vi "Single Panel - Insert VI - Subpanel.vi"(11 "VI Name":string) -> ()   [LabVIEW 2014]
uses:
  <vilib>/Utility/miscctls.llb/LVPositionTypeDef.ctl
  <vilib>/Utility/miscctls.llb/LVBoundsTypeDef.ctl
  VI Data.ctl
  Panel Data.ctl
  <vilib>/Utility/miscctls.llb/LVPointTypeDef.ctl
  Panel Global Methods.ctl
  Sub Function/Windows Utilities/Controls/Window Rectangle.ctl
  Sub Function/Windows Utilities/WinUtil HWND/Get Window HWnd.vi
  Sub Function/Windows Utilities/WinUtil HWND/Get Window Rectangle (hwnd).vi
  Sub Function/Windows Utilities/WinUtil HWND/Window Style/Set Window GWL_Style.vi
  <userlib>/_OpenG.lib/error/error.llb/Build Error Cluster__ogtk.vi
  Sub Function/Windows Utilities/WinUtil HWND/Window Style/Modify Window Style.vi
  <userlib>/_OpenG.lib/file/file.llb/Strip Path Extension - String__ogtk.vi
panel:
  in  "Dock Event":refnum<user-event>
  in  "Events Registered":T1
  in  "Move Event":refnum<user-event>
  in  "error in (no error)":errorcluster
  in  "Menu":bool
  in  "Pane Offset":T2={"Left"=0, "Top"=22}
  in  "User Events VR":variant
  out "error out":errorcluster
  in  "Title":string
  in  "Undock":bool
  in  "Expand":bool
  in  "Containing Pane":refnum<vi>
  out "2D Picture":picture
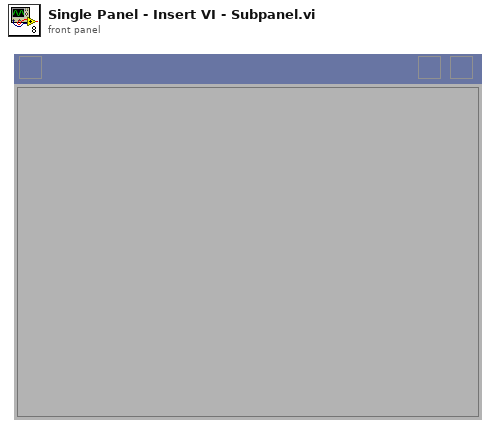
[diagram p1: front panel]
types:
  T1 = typedef "Semaphore RefNum" = refnum<k1>
  T2 = typedef "LVPositionTypeDef.ctl" = cluster{"Left":i32, "Top":i32}
  T3 = typedef "Panel Data.ctl" = cluster{"Panel VI Name":string, "Hwnd":u32, "Collapsed?":bool, "Panel Ref":refnum<vi>, "Events Variant":variant, "Resizeable?":bool, "Un-Dockedable?":bool, "Docked?":bool}
  T4 = typedef "VI Data.ctl" = cluster{"VI Name":string, "VI Ref":refnum<vi>, "Events Variant":variant, "Panel Settings":variant}
  T5 = typedef "LVBoundsTypeDef.ctl" = cluster{"Width":u32, "Height":u32}
  T6 = cluster{"Event Ref":refnum<event-registration>, "Reposition Offset":cluster{"Left":i16, "Top":i32}, "Saved Panel Size":T5, "Sub Panel":refnum<vi>, "VI Data":T4, "Panel Data":T3, "Reply User Event":refnum<user-event>, "Parent Hwnd":u32, "Parent Pane":refnum<vi>, "Pane Offset":T2, "Currently Resizeable?":bool, "Move Event":refnum<user-event>, "Dock Event":refnum<user-event>}
  T7 = typedef "LVPointTypeDef.ctl" = cluster{"Horizontal":i16, "Vertical":i16}
  T8 = enum8{"Enabled", "Disabled", "Disabled and Grayed Out"}
  T9 = typedef "Panel Global Methods.ctl" = enum16{"Read All Panels", "Read Panel Data", "Write Panel Data"}
  T10 = typedef "Window Rectangle.ctl" = cluster{"left":i16, "top":i16, "right":i16, "bottom":i16}
  T11 = enum16{"Clear Error And Continue", "Notify User Clear Error", "Clear Error Cleanup"}
  T12 = typedef "LVRectTypeDef.ctl" = cluster{"Left":i16, "Top":i16, "Right":i16, "Bottom":i16}
  T13 = typedef "Window Rectangle (hwnd).ctl" = cluster{"left":i16, "top":i16, "right":i16, "bottom":i16}
  T14 = typedef "imagedata.ctl" = cluster{"image type":i32, "image depth":i32, "image":u8[], "mask":u8[], "colors":u32[], "Rectangle":cluster{"left":i16, "top":i16, "right":i16, "bottom":i16}}
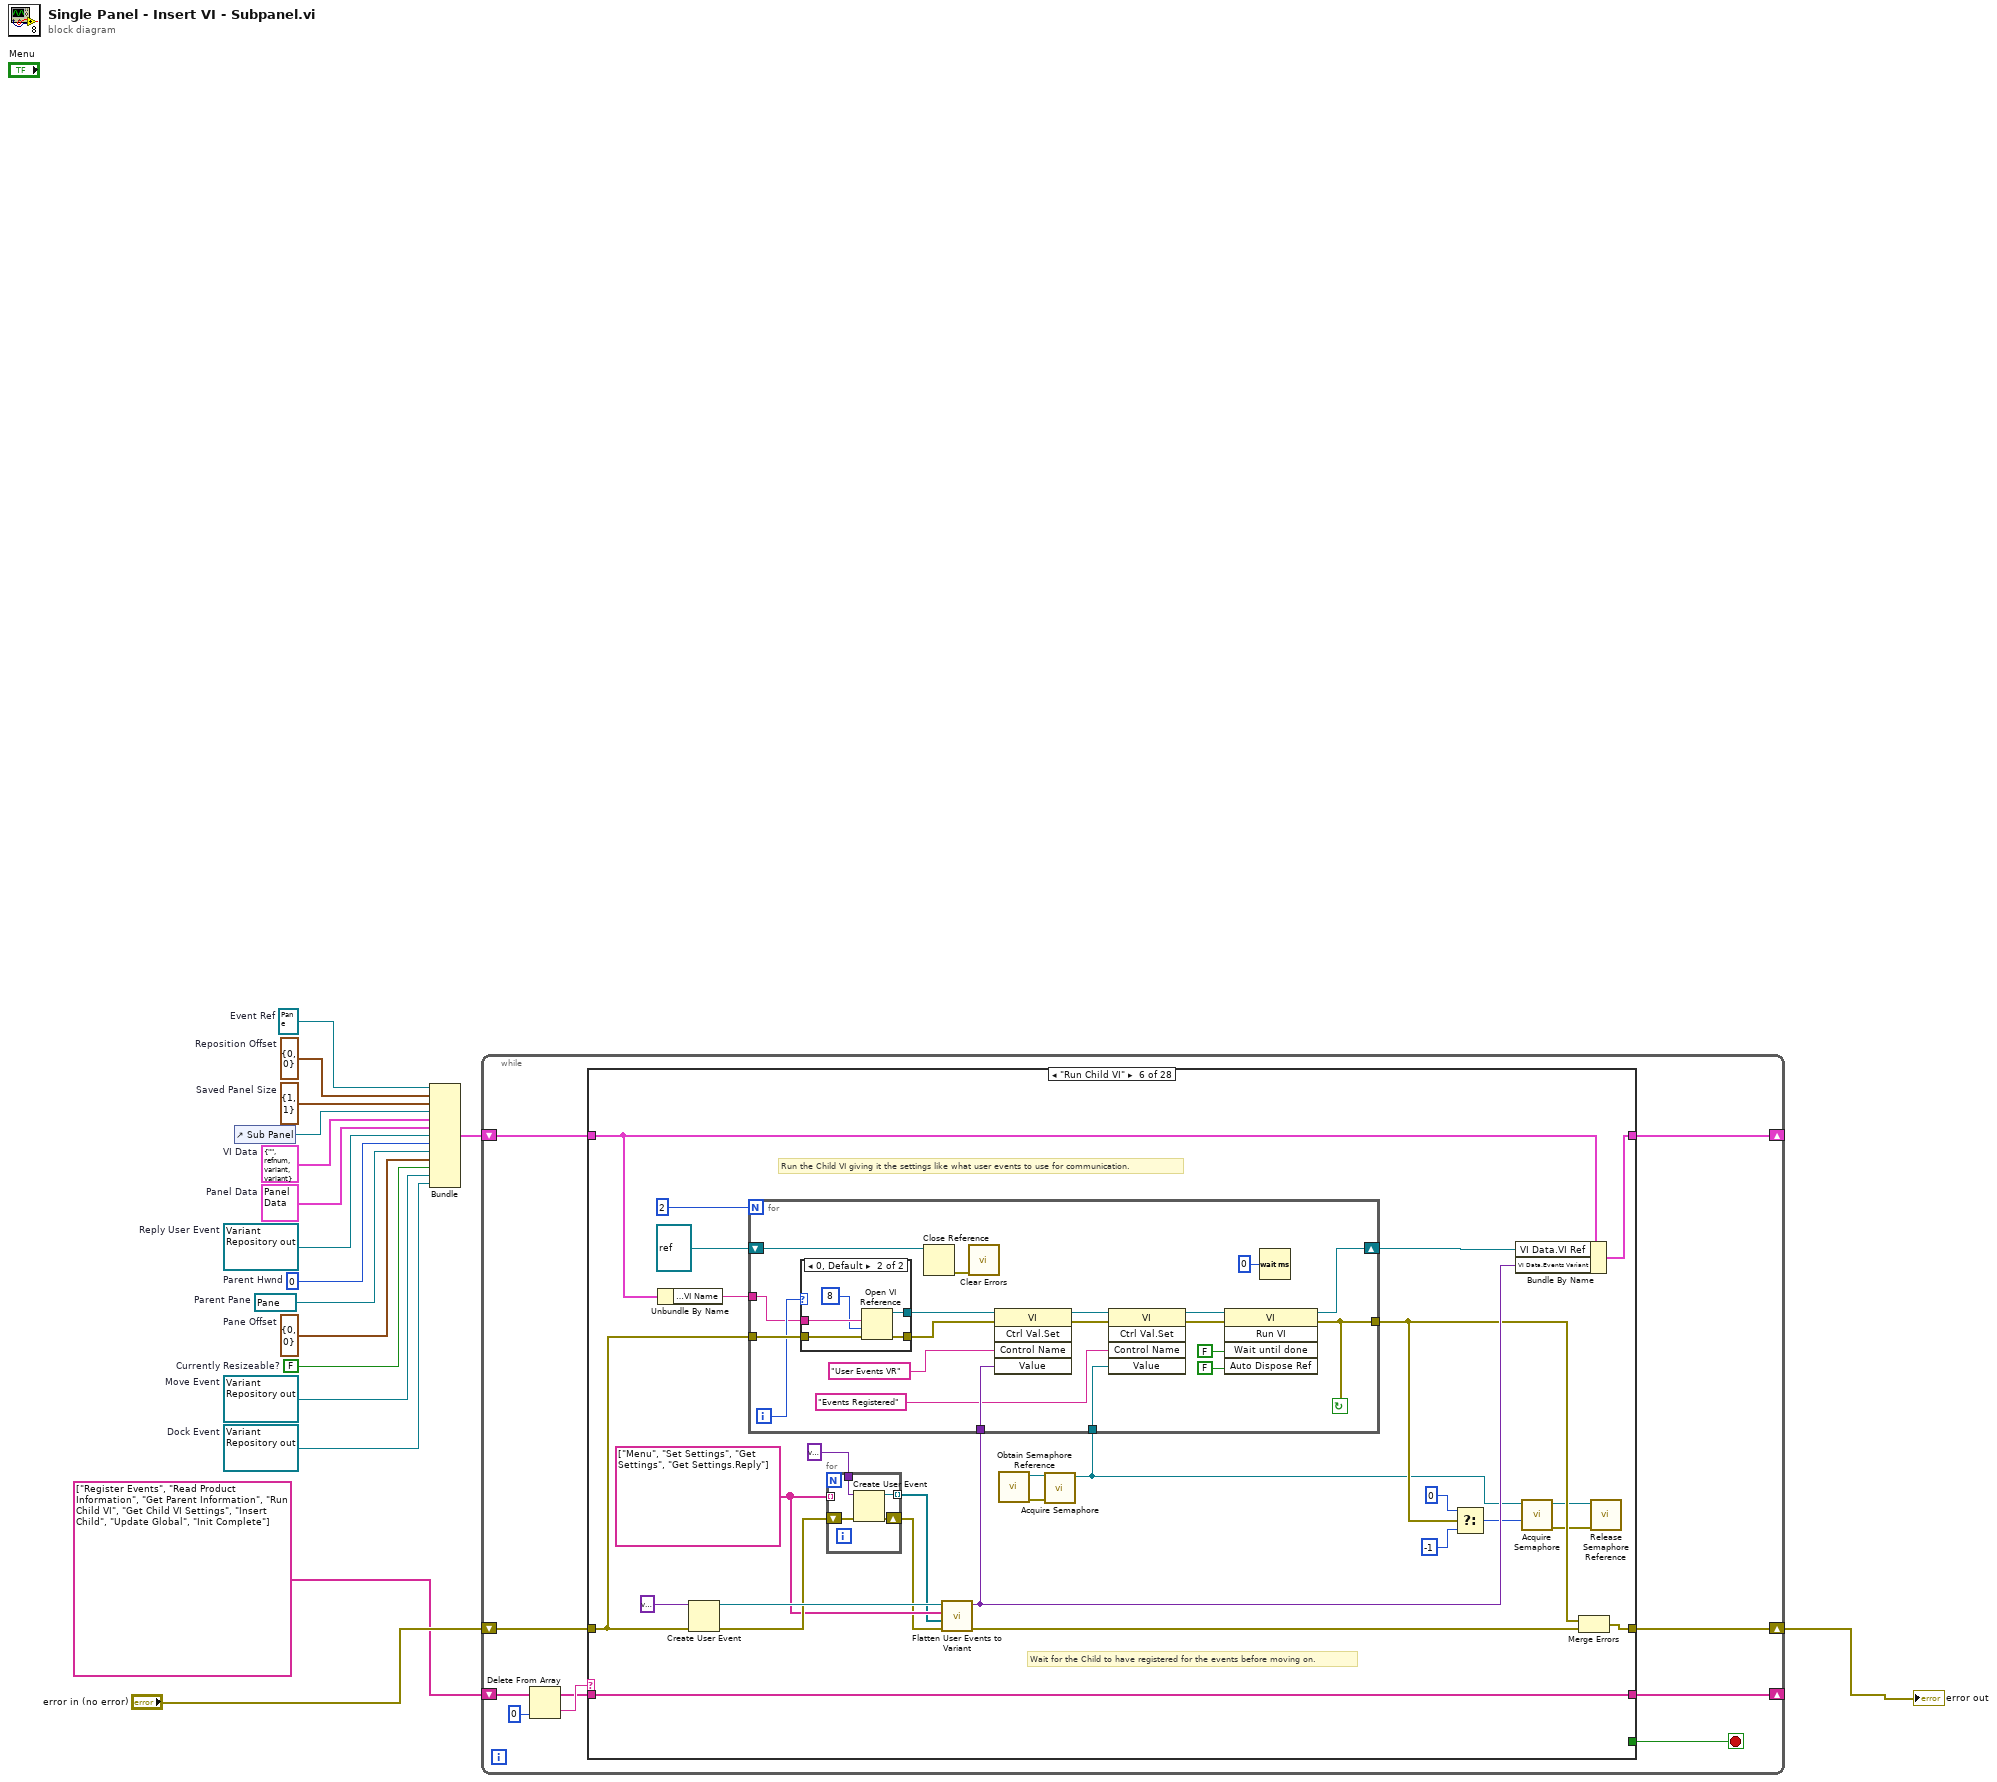
[diagram p0: block diagram]
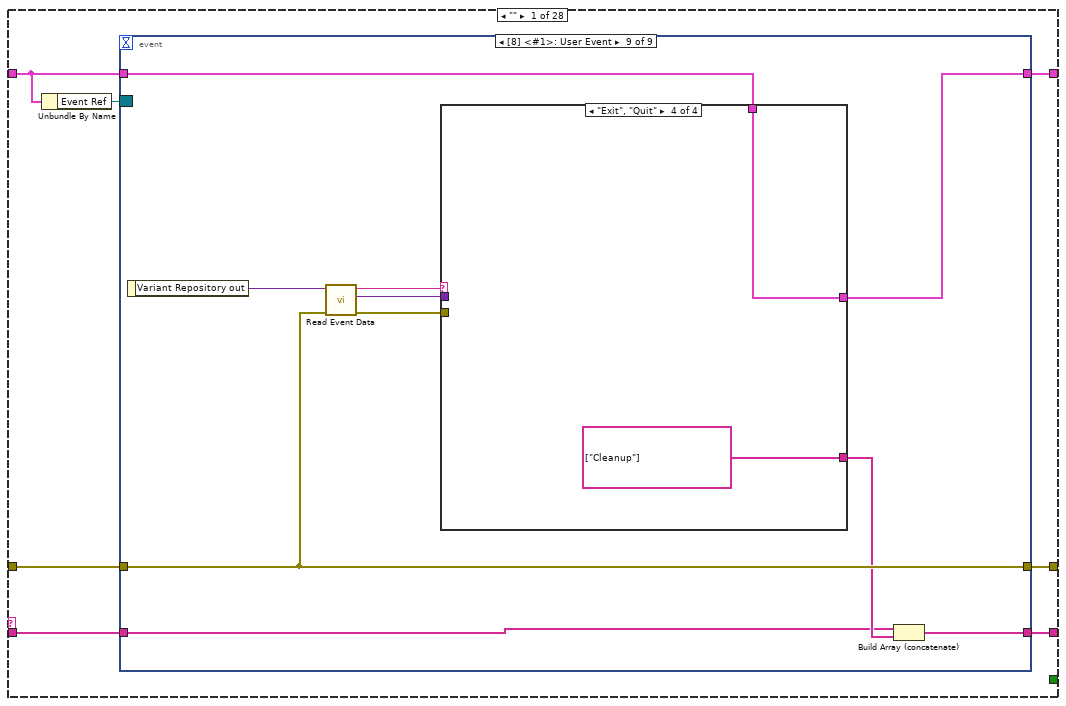
[diagram p2: hidden frame]
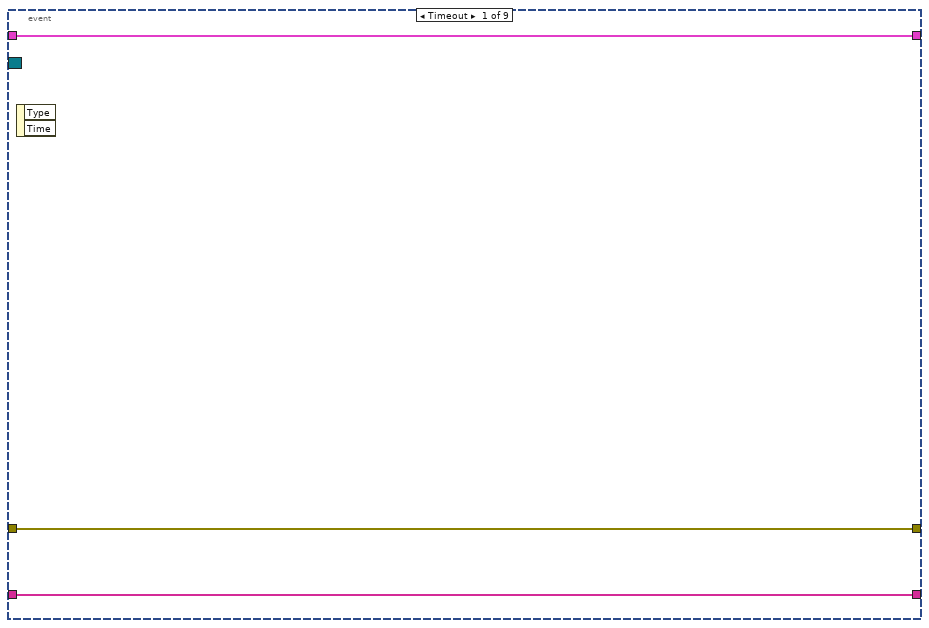
[diagram p3: hidden frame]
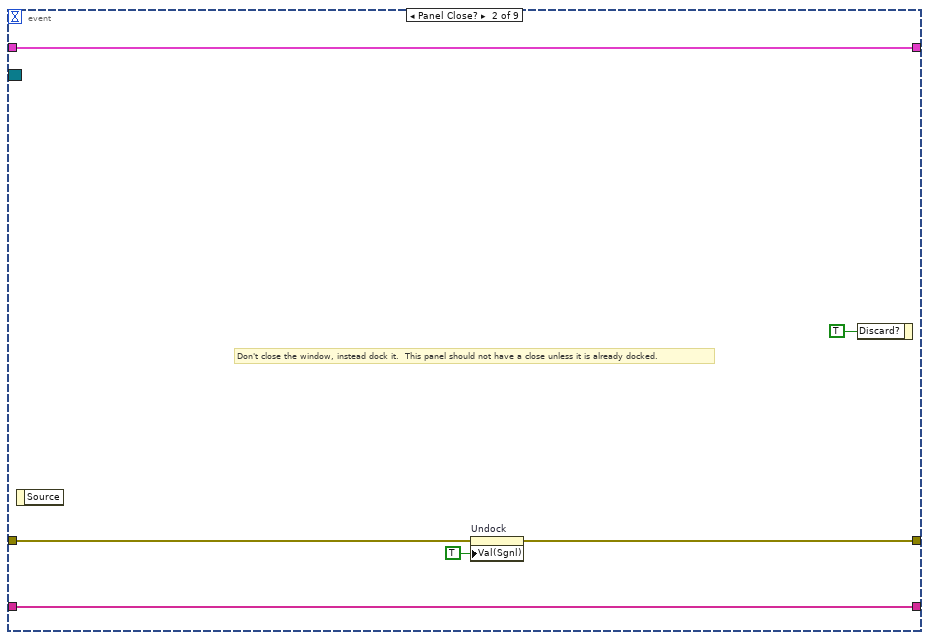
[diagram p4: hidden frame]
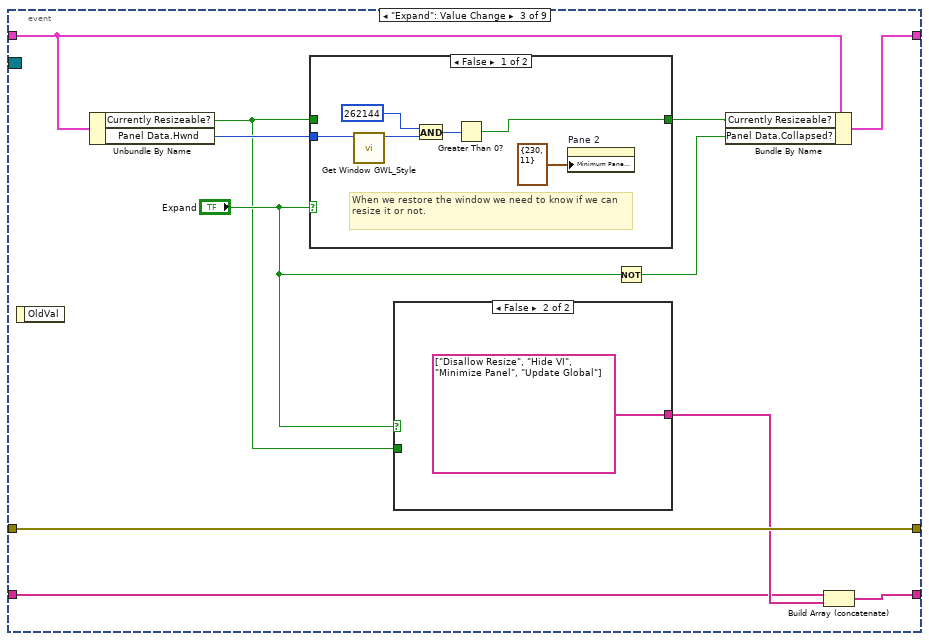
[diagram p5: hidden frame]
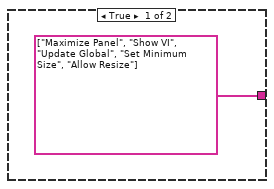
[diagram p6: hidden frame]
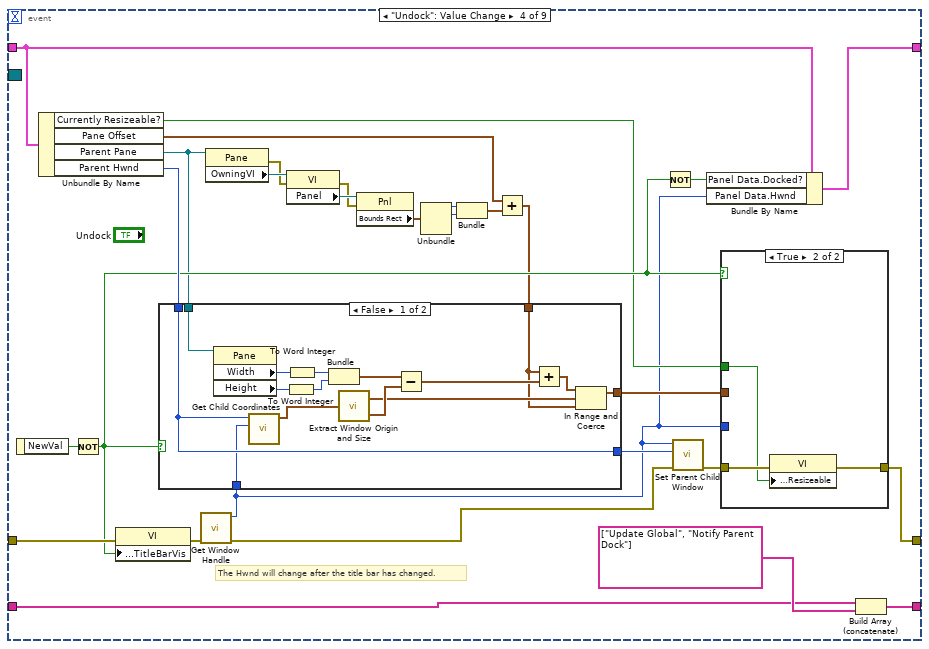
[diagram p8: hidden frame]
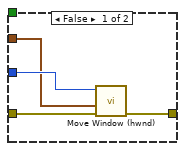
[diagram p9: hidden frame]
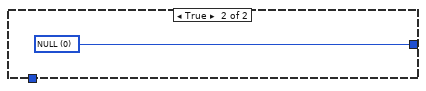
[diagram p10: hidden frame]
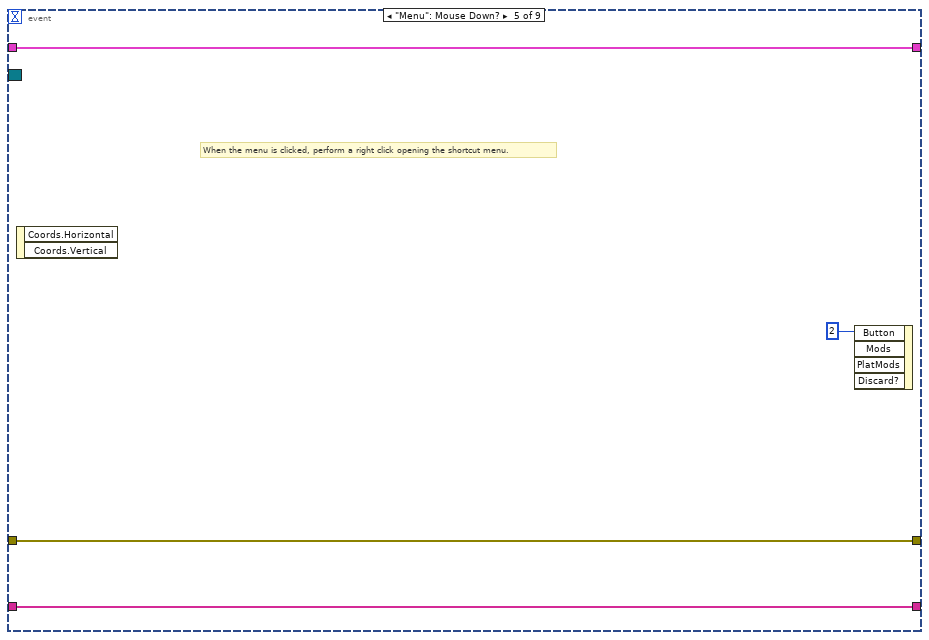
[diagram p11: hidden frame]
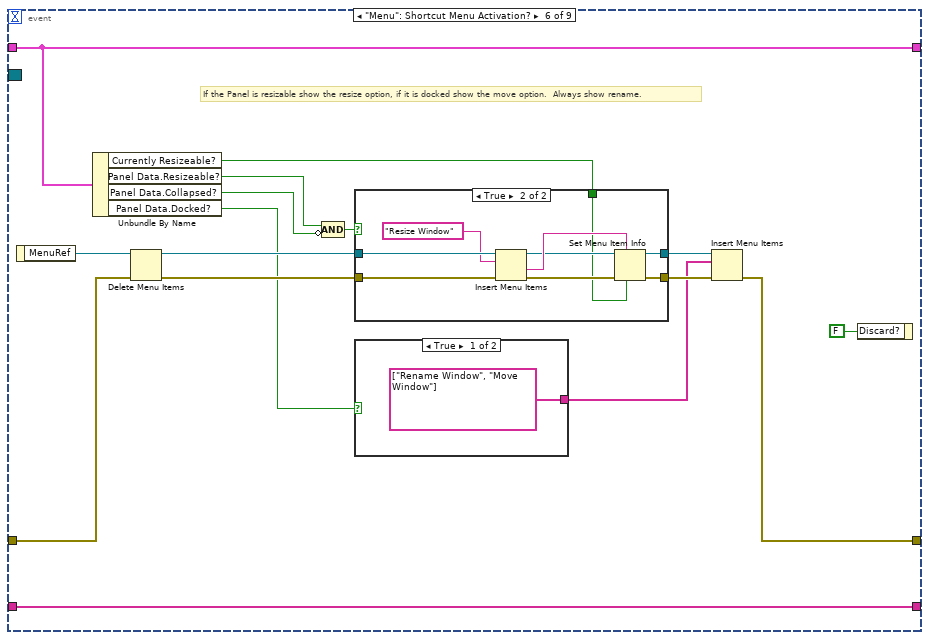
[diagram p12: hidden frame]
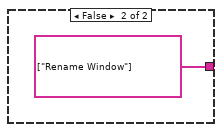
[diagram p13: hidden frame]
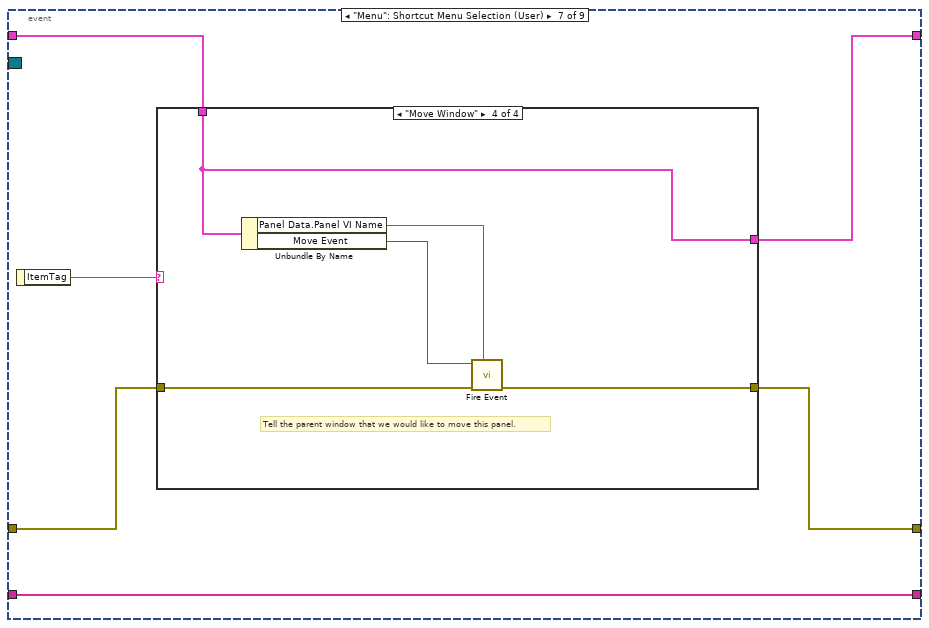
[diagram p15: hidden frame]
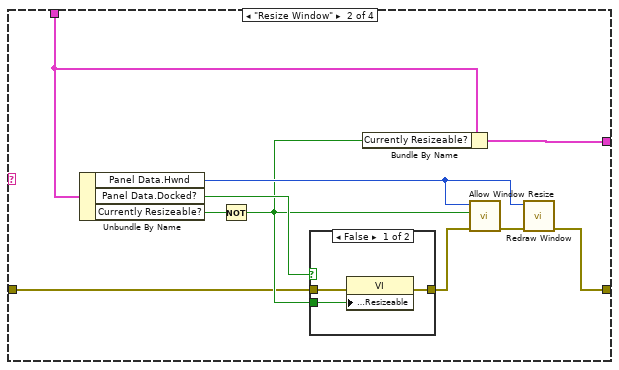
[diagram p17: hidden frame]
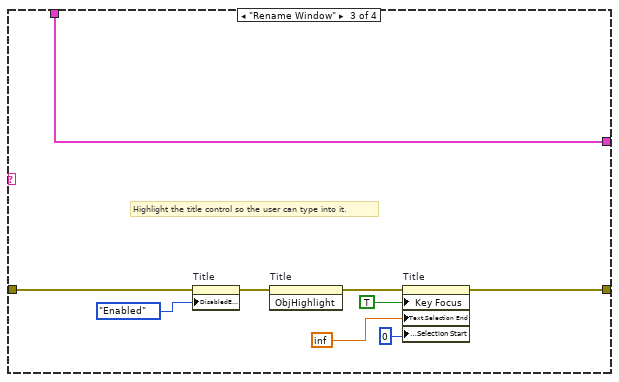
[diagram p19: hidden frame]
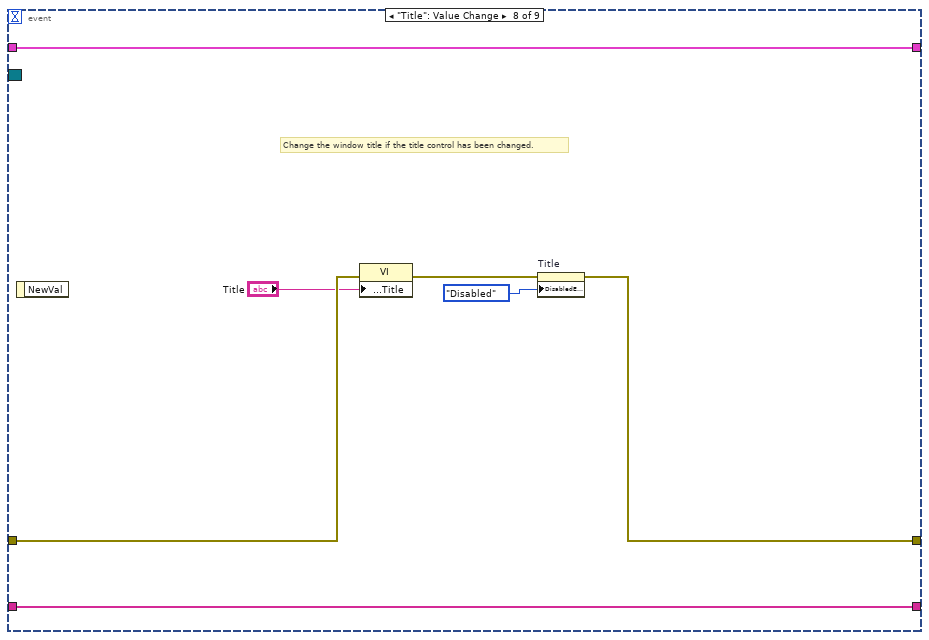
[diagram p20: hidden frame]
diagram:
  w3 = refnum<user-event> refnum  # Dock Event
  w4 = refnum<user-event> refnum  # Move Event
  w5 = FALSE  # Currently Resizeable?
  w6 = T2 {"Left"=0, "Top"=0}  # Pane Offset
  w7 = refnum<vi> refnum  # Parent Pane
  w8 = u32 0  # Parent Hwnd
  w9 = refnum<user-event> refnum  # Reply User Event
  w10 = refnum<event-registration> refnum  # Event Ref
  w11 = T3 {"Panel VI Name"="", "Hwnd"=0, "Collapsed?"=FALSE, "Panel Ref"=refnum, "Events Variant"=variant, "Resizeable?"=FALSE, "Un-Dockedable?"=FALSE, "Docked?"=FALSE}  # Panel Data
  w12 = T4 {"VI Name"="", "VI Ref"=refnum, "Events Variant"=variant, "Panel Settings"=variant}  # VI Data
  w14 = T5 {"Width"=1, "Height"=1}  # Saved Panel Size
  w15 = cluster{"Left":i16, "Top":i32} {"Left"=0, "Top"=0}  # Reposition Offset
  n1 = control-ref of="Sub Panel"() -> (w13:refnum<vi>)
  n2 = Bundle("Event Ref"=w10, "Reposition Offset"=w15, "Saved Panel Size"=w14, "Sub Panel"=w13, "VI Data"=w12, "Panel Data"=w11, "Reply User Event"=w9, "Parent Hwnd"=w8, "Parent Pane"=w7, "Pane Offset"=w6, "Currently Resizeable?"=w5, "Move Event"=w4, "Dock Event"=w3) -> (w17:T6)  [unwired: 1 in]
  n3 = while {
    shift-right: [w23] -> w2
    shift-left: "error in (no error)" -> [w27]
    shift-right: [w25] -> _
    shift-left: w17 -> [w26]
    shift-right: [w18] -> _
    shift-left: string[] ["Register Events", "Read Product Information", "Get Parent Information", "Run Child VI", "Get Child VI Settings", "Insert Child", "Update Global", "Init Complete"] ("Initialized States") -> [w19]
    stop <- w24 stop-if-true
    n4 = Delete From Array(array=w19, index=0) -> (deleted portion=w21:string, array with subset deleted=w20:string[])  [unwired: 1 in]
    n5 = case "State Machine" shown="\"Run Child VI\"" w21 {
      selector: w21 -> [_ _ _ _ _ _ _ _ _ _ _ _ _ _ _ _ w466 w477 _ _ _ _ w589 _ _ _ _ _]
      tunnel: w20 -> [w34 w212 w244 w263 w282 w309 w344 w367 w376 w394 w402 w404 w419 w426 w447 w457 w470 w481 w548 w555 w567 w569 w593 w596 w598 w611 w616 w620]
      tunnel: [w30 w212 w244 w263 w282 w309 w343 w367 w376 w394 w402 w403 w419 w426 w447 w457 w470 w481 w548 w555 w567 w570 w593 w596 w597 w611 w616 w620] -> w18
      tunnel: [w31 w210 w232 w247 w266 w303 w350 w356 w372 w377 w396 w408 w418 w425 w431 w448 w462 w506 w544 w550 w566 w571 w586 w595 w601 w603 w612 w617] -> w23
      tunnel: w27 -> [w32 w210 w226 w248 w264 w290 w351 w357 w375 w387 w397 w409 w418 w422 w435 w450 w460 w506 w545 w551 w566 w572 w587 w595 w601 w605 w613 w617]
      tunnel: w26 -> [w29 w211 w243 w262 w281 w305 w355 w366 w374 w393 w401 w411 w417 w423 w446 w454 w468 w476 w547 w552 w565 w573 w592 w594 w600 w608 w615 w619]
      tunnel: [w33 w211 w234 w257 w277 w306 w354 w366 w374 w383 w401 w407 w417 w423 w446 w452 w468 w475 w547 w552 w565 w573 w592 w594 w600 w608 w615 w619] -> w25
      tunnel: [_ _ _ _ _ _ _ _ _ _ _ _ _ _ _ _ _ _ _ _ _ _ _ _ _ _ _ TRUE] -> w24
      frame "" {
        n6 = Unbundle By Name(w29) -> ("Event Ref"=w28:refnum<event-registration>)
        n7 = event shown="[8] <#1>: User Event" {
          selector: w28 -> [_ _ _ _ _ _ _ _ _]
          dyn-events: _ -> [_ _ _ _ _ _ _ _ _]
          timeout: _ -> [_ _ _ _ _ _ _ _ _]
          tunnel: w29 -> [w37 w41 w52 w92 w119 w130 w151 w188 w195]
          tunnel: w34 -> [w35 w42 w45 w65 w117 w135 w154 w190 w192]
          tunnel: [w37 w41 w53 w85 w119 w130 w153 w188 w194] -> w33
          tunnel: w32 -> [w36 w39 w54 w91 w118 w122 w150 w186 w199]
          tunnel: [w36 w38 w54 w84 w118 w121 w149 w185 w199] -> w31
          tunnel: [w35 w42 w44 w64 w117 w135 w154 w190 w191] -> w30
          event Timeout {
            n8 = event-data() -> ()  [unwired: 1 in, 2 out]
          }
          event Panel Close? {
            # "Don't close the window, instead dock it.  This panel should not have a close unless it is already docked."
            n9 = event-data() -> ()  [unwired: 1 in, 1 out]
            n10 = property on="Undock" class="Bool (strict)"(error in=w39, "Val(Sgnl)"=TRUE ("Value (Signaling)")) -> (error out=w38:errorcluster)  [unwired: 1 in, 1 out]
            n11 = event-data("Discard?"=TRUE) -> ()  [unwired: 1 in, 1 out]
          }
          event "Expand": Value Change {
            n12 = event-data() -> ()  [unwired: 1 in, 1 out]
            n13 = Unbundle By Name(w52) -> ("Currently Resizeable?"=w47:bool, "Panel Data.Hwnd"=w50:u32)
            n14 = case shown="False" "Expand" {
              tunnel: w50 -> [w61 _]
              tunnel: [w57 w63] -> w49
              tunnel: w47 -> [_ w63]
              frame False {
                # "When we restore the window we need to know if we can resize it or not."
                n15 = call "Get Window GWL_Style.vi"("Hwnd"=w61) -> ("Style"=w60:u32)  [unwired: 9 in, 1 out]
                n16 = And(x=u32 262144 ("Value"), y=w60) -> (x .and. y?=w58:u32)
                n17 = Greater Than 0?(x=w58) -> (x > 0?=w57:bool)
                n18 = property on="Pane 2" class="Pane"("Minimum Pane Size"=T7 {"Horizontal"=230, "Vertical"=11}) -> ()  [unwired: 2 in, 2 out]
              }
              frame True {
              }
            }
            n19 = case shown="False" "Expand" {
              tunnel: [string[] ["Maximize Panel", "Show VI", "Update Global", "Set Minimum Size", "Allow Resize"] ("Elements to Add") string[] ["Disallow Resize", "Hide VI", "Minimize Panel", "Update Global"] ("Elements to Add")] -> w46
              tunnel: w47 -> [_ _]
              frame True {
              }
              frame False {
              }
            }
            n20 = Not(x="Expand") -> (.not. x?=w48:bool)
            n21 = Bundle By Name(cluster=w52, "Currently Resizeable?"=w49, "Panel Data.Collapsed?"=w48) -> (w53:T6)
            n22 = Build Array (concatenate)(w45, w46) -> (w44:string[])
          }
          event "Undock": Value Change {
            # "The Hwnd will change after the title bar has changed."
            n23 = event-data() -> ("NewVal"=w88:bool)  [unwired: 1 in]
            n24 = Unbundle By Name(w92) -> ("Currently Resizeable?"=w79:bool, "Pane Offset"=w71:T2, "Parent Pane"=w78:refnum<vi>, "Parent Hwnd"=w89:u32)
            n25 = Not(x=w88) -> (.not. x?=w82:bool)
            n26 = property class="VI"(error in=w91, "Front Panel.TitleBarVis"=w82) -> (error out=w87:errorcluster)  [unwired: 1 in, 1 out]
            n27 = call "Get Window Handle.vi"("error in (no error)"=w87) -> ("error out"=w86:errorcluster, "HWnd Out"=w67:u32)  [unwired: 9 in]
            n28 = property class="Pane"(reference=w78) -> (error out=w69:errorcluster, "OwningVI"=w77:refnum<vi>)  [unwired: 1 in, 1 out]
            n29 = property class="VI"(reference=w77, error in=w69) -> (error out=w68:errorcluster, "Panel"=w76:refnum<vi>)  [unwired: 1 out]
            n30 = property class="Pnl"(reference=w76, error in=w68) -> ("Bounds Rect"=w75:T12)  [unwired: 2 out]
            n31 = Unbundle(w75) -> ("Left"=w74:i16, "Top"=w73:i16)  [unwired: 2 out]
            n32 = Bundle("Left"=w74, "Top"=w73) -> (w72:cluster{"Left":i16, "Top":i16})  [unwired: 1 in]
            n33 = Add(x=w71, y=w72) -> (x+y=w70:T2)
            n34 = case shown="False" w82 {
              tunnel: [w111 w115] -> w80
              tunnel: w89 -> [w111 _]
              tunnel: [w104 _] -> w83
              tunnel: w67 -> [w110 _]
              tunnel: w78 -> [w109 _]
              tunnel: w70 -> [w100 _]
              frame False {
                n35 = property class="Pane"(reference=w109) -> ("Width"=w108:u32, "Height"=w107:u32)  [unwired: 1 in, 2 out]
                n36 = call "Get Child Coordinates.vi"("Child hWnd"=w110, "Parent hWnd"=w111) -> ("Relative"=w114:T13)  [unwired: 7 in, 2 out]
                n37 = To Word Integer(number=w107) -> (16bit integer=w102:i16)
                n38 = To Word Integer(number=w108) -> (16bit integer=w103:i16)
                n39 = Bundle(w103, w102) -> (w112:cluster{i16, i16})  [unwired: 1 in]
                n40 = call "Extract Window Origin and Size.vi"("window rect"=w114) -> ("window origin"=w106:cluster{"left":i16, "top":i16}, "window size"=w113:cluster{"width":i16, "height":i16})
                n41 = Subtract(x=w112, y=w113) -> (x-y=w105:cluster{i16, i16})
                n42 = Add(x=w100, y=w105) -> (x+y=w101:T2)
                n43 = In Range and Coerce(upper limit=w101, x=w106, lower limit=w100) -> (coerced(x)=w104:T2)  [unwired: 1 out]
              }
              frame True {
                w115 = u32 0 items=["NULL"]
              }
            }
            n44 = Not(x=w82) -> (.not. x?=w81:bool)
            n45 = call "Set Parent Child Window.vi"("error in (no error)"=w86, "new parent"=w80, "child"=w67) -> ("error out"=w90:errorcluster)  [unwired: 8 in]
            n46 = Bundle By Name(cluster=w92, "Panel Data.Docked?"=w81, "Panel Data.Hwnd"=w67) -> (w85:T6)
            n47 = case shown="True" w82 {
              tunnel: w90 -> [w96 w99]
              tunnel: [w95 w98] -> w84
              tunnel: w67 -> [w94 _]
              tunnel: w83 -> [w93 _]
              tunnel: w79 -> [_ w97]
              frame False {
                n48 = call "Move Window (hwnd).vi"("error in (no error)"=w96, "New Position (0,0)"=w93, "HWnd"=w94) -> ("error out"=w95:errorcluster)  [unwired: 6 in, 2 out]
              }
              frame True {
                n49 = property class="VI"(error in=w99, "Front Panel.Resizeable"=w97) -> (error out=w98:errorcluster)  [unwired: 1 in, 1 out]
              }
            }
            n50 = Build Array (concatenate)(w65, string[] ["Update Global", "Notify Parent Dock"]) -> (w64:string[])
          }
          event "Menu": Mouse Down? {
            # "When the menu is clicked, perform a right click opening the shortcut menu."
            n51 = event-data() -> ()  [unwired: 1 in, 2 out]
            n52 = event-data("Button"=u16 2) -> ()  [unwired: 4 in, 1 out]
          }
          event "Menu": Shortcut Menu Activation? {
            # "If the Panel is resizable show the resize option, if it is docked show the move option.  Always show rename."
            n53 = event-data() -> ("MenuRef"=w134:refnum<k9>)  [unwired: 1 in]
            n54 = Unbundle By Name(w130) -> ("Currently Resizeable?"=w129:bool, "Panel Data.Resizeable?"=w128:bool, "Panel Data.Collapsed?"=w126:bool, "Panel Data.Docked?"=w120:bool)
            n55 = Delete Menu Items(6:w122, 9:w134) -> (0:w132:errorcluster, 3:w133:refnum<k9>)  [unwired: 2 in]
            n56 = Compound Arithmetic op=AND(w128, invert w126) -> (w127:bool)
            n57 = case shown="True" w127 {
              tunnel: w133 -> [w139 w148]
              tunnel: w132 -> [w138 w147]
              tunnel: w129 -> [_ w142]
              tunnel: [w138 w141] -> w125
              tunnel: [w139 w140] -> w124
              frame False {
              }
              frame True {
                n58 = Insert Menu Items(6:w147, 8:"Resize Window", 9:w148) -> (0:w144:errorcluster, 1:w145:string, 3:w143:refnum<k9>)  [unwired: 3 in]
                n59 = Set Menu Item Info(6:w142, 7:w145, 8:w144, 11:w143) -> (0:w141:errorcluster, 3:w140:refnum<k9>)  [unwired: 3 in]
              }
            }
            n60 = case shown="True" w120 {
              tunnel: [string[] ["Rename Window", "Move Window"] string[] ["Rename Window"]] -> w123
              frame True {
              }
              frame False {
              }
            }
            n61 = Insert Menu Items(6:w125, 8:w123, 9:w124) -> (0:w121:errorcluster)  [unwired: 3 in, 2 out]
            n62 = event-data("Discard?"=FALSE) -> ()  [unwired: 1 in, 1 out]
          }
          event "Menu": Shortcut Menu Selection (User) {
            n63 = event-data() -> ("ItemTag"=w152:string)  [unwired: 1 in]
            n64 = case shown="\"Move Window\"" w152 {
              tunnel: [w156 w162 w172 w179] -> w153
              tunnel: w151 -> [w156 w159 w172 w179]
              tunnel: w150 -> [w155 w158 w171 w181]
              tunnel: [w155 w157 w170 w180] -> w149
              frame Default {
              }
              frame "Resize Window" {
                n65 = Unbundle By Name(w159) -> ("Panel Data.Hwnd"=w165:u32, "Panel Data.Docked?"=w163:bool, "Currently Resizeable?"=w161:bool)
                n66 = Not(x=w161) -> (.not. x?=w160:bool)
                n67 = case shown="False" w163 {
                  tunnel: [w169 _] -> w164
                  tunnel: w160 -> [w168 _]
                  tunnel: w158 -> [w167 _]
                  frame False {
                    n68 = property class="VI"(error in=w167, "Front Panel.Resizeable"=w168) -> (error out=w169:errorcluster)  [unwired: 1 in, 1 out]
                  }
                  frame True {
                  }
                }
                n69 = Bundle By Name(cluster=w159, "Currently Resizeable?"=w160) -> (w162:T6)
                n70 = call "Allow Window Resize.vi"("error in (no error)"=w164, "Allow Resize?"=w160, "Hwnd"=w165) -> ("error out"=w166:errorcluster)  [unwired: 8 in]
                n71 = call "Redraw Window.vi"("error in (no error)"=w166, "Hwnd"=w165) -> ("error out"=w157:errorcluster)  [unwired: 9 in]
              }
              frame "Rename Window" {
                # "Highlight the title control so the user can type into it."
                n72 = property on="Title" class="Str"(error in=w171, "DisabledEnum"=T8."Enabled" ("Disabled")) -> (error out=w176:errorcluster)  [unwired: 1 in, 1 out]
                n73 = invoke on="Title" class="Str" method="ObjHighlight"(error in=w176) -> (error out=w175:errorcluster)  [unwired: 2 in, 2 out]
                n74 = property on="Title" class="Str"(error in=w175, "Key Focus"=TRUE, "Text.Selection End"=inf, "Text.Selection Start"=u32 0 ("Text.Selection:Start")) -> (error out=w170:errorcluster)  [unwired: 1 in, 1 out]
              }
              frame "Move Window" {
                # "Tell the parent window that we would like to move this panel."
                n75 = Unbundle By Name(w179) -> ("Panel Data.Panel VI Name"=w182:string, "Move Event"=w183:refnum<user-event>)
                n76 = call "Fire Event.vi"("Event Name"=w182, "error in (no error)"=w181, "User Event In"=w183) -> ("error out"=w180:errorcluster)  [unwired: 7 in, 1 out]
              }
            }
          }
          event "Title": Value Change {
            # "Change the window title if the title control has been changed."
            n77 = event-data() -> ()  [unwired: 1 in, 1 out]
            n78 = property class="VI"(error in=w186, "Front Panel.Title"="Title") -> (error out=w187:errorcluster)  [unwired: 1 in, 1 out]
            n79 = property on="Title" class="Str"(error in=w187, "DisabledEnum"=T8."Disabled" ("Disabled")) -> (error out=w185:errorcluster)  [unwired: 1 in, 1 out]
          }
          event User Event {
            n80 = event-data() -> ("Variant Repository out"=w200:variant)  [unwired: 1 in]
            n81 = call "Read Event Data.vi"("error in (no error)"=w199, "Variant Data"=w200) -> ("error out"=w198:errorcluster, "Event Data"=w196:variant, "Event Name"=w197:string)  [unwired: 7 in]
            n82 = case shown="\"Exit\", \"Quit\"" w197 {
              tunnel: w198 -> [_ _ _ _]
              tunnel: [_ string[] ["Get Settings", "Send Settings to Parent"] string[] ["Set Settings"] string[] ["Cleanup"]] -> w193
              tunnel: w196 -> [_ _ w204 _]
              tunnel: w195 -> [w201 w202 w206 w208]
              tunnel: [w201 w202 w205 w208] -> w194
              frame Default {
              }
              frame "Get Settings" {
              }
              frame "Set Settings" {
                n83 = Bundle By Name(cluster=w206, "VI Data.Panel Settings"=w204) -> (w205:T6)
              }
              frame "Exit", "Quit" {
              }
            }
            n84 = Build Array (concatenate)(w192, w193) -> (w191:string[])
          }
        }
      }
      frame "----Initialize----" {
      }
      frame "Register Events" {
        n85 = Get Variant Attribute(Variant="User Events VR", name="Event Names" ("Tag"), default value (empty Variant)=string[] [], error in=w226) -> (duplicate Variant=w221:variant, value=w222:string[], error out=w220:errorcluster)  [unwired: 1 out]
        n86 = Get Variant Attribute(Variant=w221, name="User Events" ("Tag"), error in=w220) -> (duplicate Variant=w217:variant, value=w218:variant, error out=w216:errorcluster)  [unwired: 1 in, 1 out]
        n87 = Search 1D Array(1D array=w222, element="Get Settings.Reply") -> (index of element=w239:i32)  [unwired: 1 in]
        n88 = Get Variant Attribute(Variant=w217, name="Quit Event" ("Tag"), error in=w216) -> (value=w214:variant, error out=w213:errorcluster)  [unwired: 1 in, 2 out]
        n89 = Variant To Data(error in=w213, type=refnum<user-event>[] [] ("All User Events"), Variant=w218) -> (data=w238:refnum<user-event>[], error out=w229:errorcluster)
        n90 = Delete From Array(array=w238, index=w239) -> (deleted portion=w231:refnum<user-event>, array with subset deleted=w237:refnum<user-event>[])  [unwired: 1 in]
        n91 = Variant To Data(error in=w229, type=refnum<user-event> refnum ("Quit Event"), Variant=w214) -> (data=w236:refnum<user-event>, error out=w228:errorcluster)
        n92 = Build Array (concatenate)(w237, w236) -> (w235:refnum<user-event>[])
        n93 = register-events(error in=w228, w235) -> (reference out=w233:refnum<event-registration>, error out=w232:errorcluster)  [unwired: 1 in]
        n94 = Bundle By Name(cluster=w243, "Dock Event"="Dock Event", "Move Event"="Move Event", "Reply User Event"=w231, "Event Ref"=w233, "Panel Data.Events Variant"="User Events VR") -> (w234:T6)
      }
      frame "Read Product Information" {
        # "Get the name of the VI to be inserted in the subpanel.  If blank just use the Graph Panel which at the moment is the only one we have."
        n95 = property on="2D Picture" class="Pict"("Visible"=FALSE) -> ()  [unwired: 2 in, 2 out]
        n96 = local write "Undock"(TRUE ("Undock")) -> ()
        n97 = property on="Pane 2" class="Pane"("PaneColor"=u32 11776947) -> ()  [unwired: 2 in, 2 out]
        n98 = local write "Expand"(TRUE ("Expand")) -> ()
        n99 = vi-ref "Graph Child.vi"() -> (w261:refnum<vi>)
        n100 = property on="Title" class="Str"("DisabledEnum"=T8."Disabled" ("Disabled")) -> ()  [unwired: 2 in, 2 out]
        n101 = property class="VI"(reference=w261) -> ("Name"=w259:string)  [unwired: 1 in, 2 out]
        n102 = Empty String/Path?(string/path="VI Name") -> (empty?=w260:bool)
        n103 = control-ref of="This VI"() -> (w246:refnum<vi>)
        n104 = Select(t=w259, s=w260, f="VI Name") -> (s? t:f=w253:string)
        n105 = call "Get VI Name From Reference.vi"("error in (no error)"=w248, "VI Ref"=w246) -> ("error out"=w247:errorcluster, "VI Name"=w249:string)  [unwired: 8 in]
        n106 = control-ref of="This VI"() -> (w252:refnum<vi>)
        n107 = call-poly <userlib>:"Strip Path Extension__ogtk.vi"("path"=w253) -> ("root"=w251:string)  [unwired: 1 out]
        n108 = Bundle By Name(cluster=w262, "Panel Data.Panel Ref"=w252, "VI Data.VI Name"=w253, "Panel Data.Panel VI Name"=w249) -> (w257:T6)
        n109 = property class="VI"("Front Panel.Title"=w251) -> ()  [unwired: 2 in, 2 out]
        n110 = local write "Title"(w251) -> ()
      }
      frame "Get Parent Information" {
        # "Get information like the Parent HWND, and HWND of this VI (also known as the Panel VI)"
        n111 = call "Get HWnd From VI Ref.vi"("error in (no error)"=w264) -> ("error out"=w274:errorcluster, "HWnd Out"=w275:u32)  [unwired: 9 in]
        n112 = control-ref of="Splitter"() -> (w278:refnum<vi>)
        n113 = property class="Splitter"(reference=w278, error in=w274) -> (error out=w273:errorcluster, "Position"=w279:i32)  [unwired: 1 out]
        n114 = property class="Pane"(reference="Containing Pane", error in=w264) -> (error out=w270:errorcluster, "OwningVI"=w271:refnum<vi>)  [unwired: 1 out]
        n115 = Increment(x=w279) -> (x+1=w272:i32)
        n116 = call "Get HWnd From VI Ref.vi"("error in (no error)"=w270, "VI reference (calling VI)"=w271) -> ("error out"=w265:errorcluster, "HWnd Out"=w269:u32)  [unwired: 8 in]
        n117 = Bundle("left"=i16 0, w272) -> (w276:cluster{"left":i16, i32})  [unwired: 1 in]
        n118 = Merge Errors(w265, w273) -> (w266:errorcluster)
        n119 = Bundle By Name(cluster=w281, "Pane Offset"="Pane Offset", "Parent Pane"="Containing Pane", "Parent Hwnd"=w269, "Reposition Offset"=w276, "Panel Data.Hwnd"=w275) -> (w277:T6)
      }
      frame "Run Child VI" {
        w285 = string[] ["Menu", "Set Settings", "Get Settings", "Get Settings.Reply"] ("User Event Names")
        # "Run the Child VI giving it the settings like what user events to use for communication."
        # "Wait for the Child to have registered for the events before moving on."
        n120 = Unbundle By Name(w305) -> ("VI Data.VI Name"=w304:string)
        n121 = Create User Event(user event datatype=variant ("Variant"), error in=w290) -> (user event=w288:refnum<user-event>, error out=w286:errorcluster)
        n122 = for {
          shift-right: [w312] -> w284
          shift-left: w286 -> [w313]
          tunnel: variant ("Event Data") -> [w311]
          tunnel: w285 -> [_] mode=indexing
          tunnel: [w310] -> w283 mode=indexing
          n123 = Create User Event(user event datatype=w311, error in=w313) -> (user event=w310:refnum<user-event>, error out=w312:errorcluster)
        }
        n124 = call "Flatten User Events to Variant.vi"("error in (no error)"=w284, "All User Events"=w283, "All User Event Names"=w285, "Quit Event"=w288) -> ("error out"=w301:errorcluster, "Variant"=w300:variant)  [unwired: 6 in]
        n125 = call <vilib>:"Obtain Semaphore Reference.vi"() -> ("error out"=w296:errorcluster, "semaphore"=w295:T1)  [unwired: 5 in, 1 out]
        n126 = call <vilib>:"Acquire Semaphore.vi"("error in (no error)"=w296, "semaphore"=w295) -> ("semaphore out"=w291:T1)  [unwired: 3 in, 2 out]
        n127 = for {
          N: 2 -> [_]
          tunnel: w300 -> [w330]
          tunnel: w290 -> [w326]
          tunnel: [w324] -> w297
          shift-right: [w325] -> w302
          shift-left: refnum<vi> refnum ("vi reference") -> [w322]
          tunnel: w304 -> [w320]
          tunnel: w291 -> [w315]
          i -> [w323]
          stop <- w324 continue-if-true
          n128 = case shown="0, Default" w323 {
            tunnel: [w336 w342] -> w333
            tunnel: [w337 w341] -> w331
            tunnel: w320 -> [w334 w340]
            tunnel: w326 -> [w335 w339]
            frame 1 {
              n129 = Open VI Reference(vi path=w334, error in (no error)=w335) -> (vi reference=w337:refnum<vi>, error out=w336:errorcluster)  [unwired: 4 in]
            }
            frame 0, Default {
              n130 = Open VI Reference(vi path=w340, options=8, error in (no error)=w339) -> (vi reference=w341:refnum<vi>, error out=w342:errorcluster)  [unwired: 3 in]
            }
          }
          n131 = Close Reference(reference=w322) -> (error out=w321:errorcluster)  [unwired: 1 in]
          n132 = call <vilib>:"Clear Errors.vi"("error in (no error)"=w321) -> ()  [unwired: 5 in, 2 out]
          n133 = invoke class="VI" method="Ctrl Val.Set"(reference=w331, error in=w333, "Control Name"="User Events VR", "Value"=w330) -> (reference out=w317:refnum<vi>, error out=w332:errorcluster)  [unwired: 1 in, 3 out]
          n134 = invoke class="VI" method="Ctrl Val.Set"(reference=w317, error in=w332, "Control Name"="Events Registered", "Value"=w315) -> (reference out=w316:refnum<vi>, error out=w318:errorcluster)  [unwired: 1 in, 3 out]
          n135 = invoke class="VI" method="Run VI"(reference=w316, error in=w318, "Wait until done"=FALSE ("Wait Until Done"), "Auto Dispose Ref"=FALSE ("Auto Dispose Reference")) -> (reference out=w325:refnum<vi>, error out=w324:errorcluster)  [unwired: 1 in, 3 out]
          n136 = Wait (ms)(milliseconds to wait=u32 0) -> ()  [unwired: 1 out]
        }
        n137 = Select(t=0, s=w297, f=-1 ("ms timeout (-1)")) -> (s? t:f=w292:i32)
        n138 = Bundle By Name(cluster=w305, "VI Data.VI Ref"=w302, "VI Data.Events Variant"=w300) -> (w306:T6)
        n139 = call <vilib>:"Acquire Semaphore.vi"("ms timeout (-1)"=w292, "semaphore"=w291) -> ("error out"=w293:errorcluster, "semaphore out"=w294:T1)  [unwired: 3 in, 1 out]
        n140 = Merge Errors(w297, w301) -> (w303:errorcluster)
        n141 = call <vilib>:"Release Semaphore Reference.vi"("error in (no error)"=w293, "semaphore"=w294) -> ()  [unwired: 8 in, 2 out]
      }
      frame "Get Child VI Settings" {
        # "Store the settings"
        n142 = Unbundle By Name(w355) -> ("VI Data.VI Ref"=w353:refnum<vi>)
        n143 = property class="VI"(reference=w353, error in=w351) -> (error out=w350:errorcluster, "Front Panel.Resizeable"=w346:bool, "Front Panel.Closeable"=w347:bool)  [unwired: 1 out]
        n144 = property on="Undock" class="Bool (strict)"("Visible"=w347) -> ()  [unwired: 2 in, 2 out]
        n145 = Select(t="Allow Resize" ("String"), s=w346, f="Disallow Resize" ("String")) -> (s? t:f=w345:string)
        n146 = Bundle By Name(cluster=w355, "Panel Data.Resizeable?"=w346, "Panel Data.Un-Dockedable?"=w347, "Panel Data.Docked?"=TRUE, "Currently Resizeable?"=w346) -> (w354:T6)
        n147 = Build Array (concatenate)(w344, w345) -> (w343:string[])
      }
      frame "Insert Child" {
        w365 = FALSE ("Front Panel Window:Title Bar Visible")
        # "Insert the Child VI into the sub panel."
        n148 = Unbundle By Name(w366) -> ("Sub Panel"=w361:refnum<vi>, "VI Data.VI Ref"=w363:refnum<vi>)
        n149 = property on="Property Node" class="SubPnl"(reference=w361, error in=w357, "Visible"=TRUE) -> (reference out=w360:refnum<vi>, error out=w358:errorcluster)
        n150 = invoke on="Invoke Node" class="SubPnl" method="FitControlToPane"(reference=w360, error in=w358) -> (error out=w359:errorcluster)  [unwired: 1 in, 2 out]
        n151 = property class="VI"(reference=w363, error in=w359, "Front Panel.TitleBarVis"=w365, "Front Panel.ShowMenuBar"=w365) -> (error out=w364:errorcluster)  [unwired: 1 out]
        n152 = invoke on="Sub Panel" class="SubPanel" method="Insert VI"(error in=w364, "VI Ref"=w363) -> (error out=w356:errorcluster)  [unwired: 2 in, 3 out]
      }
      frame "Set Settings" {
        w369 = "Set Settings" ("Event Name (Quit)")
        # "Take the settings for the Child VI and send them down using the user event."
        n153 = Unbundle By Name(w374) -> ("VI Data.Panel Settings"=w368:variant, "VI Data.Events Variant"=w373:variant)
        n154 = call "Get User Event from Event Name.vi"("error in (no error)"=w375, "Event Data"=w373, "Event Name (Quit)"=w369) -> ("error out"=w371:errorcluster, "User Event out"=w370:refnum<user-event>)  [unwired: 7 in]
        n155 = call "Fire Event.vi"("Event Name"=w369, "error in (no error)"=w371, "Event Data"=w368, "User Event In"=w370) -> ("error out"=w372:errorcluster)  [unwired: 6 in, 1 out]
      }
      frame "Get Settings" {
        w388 = "Get Settings" ("Event Name (Quit)")
        # "Register for the reply before sending the request."
        # "Wait for the Child VI to send the settings back."
        # "Send the vent to get the settings from the Child VI."
        n156 = Unbundle By Name(w393) -> ("VI Data.Events Variant"=w390:variant)
        n157 = call "Get User Event from Event Name.vi"("error in (no error)"=w387, "Event Data"=w390, "Event Name (Quit)"=w388) -> ("error out"=w392:errorcluster, "User Event out"=w391:refnum<user-event>)  [unwired: 7 in]
        n158 = call "Get User Event from Event Name.vi"("error in (no error)"=w387, "Event Data"=w390, "Event Name (Quit)"="Get Settings.Reply") -> ("error out"=w384:errorcluster, "User Event out"=w382:refnum<user-event>)  [unwired: 7 in]
        n159 = register-events(error in=w384, w382) -> (reference out=w381:refnum<event-registration>, error out=w385:errorcluster)  [unwired: 1 in]
        n160 = Merge Errors(w392, w385) -> (w386:errorcluster)
        n161 = call "Fire Event.vi"("Event Name"=w388, "error in (no error)"=w386, "User Event In"=w391) -> ("error out"=w378:errorcluster)  [unwired: 7 in, 1 out]
        n162 = event shown="[0] <User Event out>: User Event" {
          selector: w381 -> [_]
          dyn-events: _ -> [_]
          timeout: _ -> [_]
          tunnel: [w395] -> w380
          event User Event {
            n163 = event-data() -> ("Variant Repository out"=w395:variant)  [unwired: 1 in]
          }
        }
        n164 = call "Read Event Data.vi"("error in (no error)"=w378, "Variant Data"=w380) -> ("error out"=w377:errorcluster, "Event Data"=w379:variant)  [unwired: 7 in, 1 out]
        n165 = Bundle By Name(cluster=w393, "VI Data.Panel Settings"=w379) -> (w383:T6)
      }
      frame "Send Settings to Parent" {
        # "Send the settings we got from the Child back up to the Parent."
        n166 = Unbundle By Name(w401) -> ("Panel Data.Panel VI Name"=w398:string, "Reply User Event"=w400:refnum<user-event>, "VI Data.Panel Settings"=w399:variant)
        n167 = call "Fire Event.vi"("Event Name"=w398, "error in (no error)"=w397, "Event Data"=w399, "User Event In"=w400) -> ("error out"=w396:errorcluster)  [unwired: 6 in, 1 out]
      }
      frame "Init Complete" {
        # "After init is complete we will tell the window to be resizeable or not.  This can't be done until the UI is showing and has an Hwnd.  Keep trying to get a HWND until one is given."
        n168 = while {
          tunnel: [w414] -> w406
          stop <- w413 stop-if-true
          n169 = call "Get Window Handle.vi"() -> ("error out"=w412:errorcluster, "HWnd Out"=w414:u32)  [unwired: 10 in]
          n170 = Wait (ms)(milliseconds to wait=u32 10) -> ()  [unwired: 1 out]
          n171 = Not Equal To 0?(x=w414) -> (x != 0?=w416:bool)
          n172 = Or(x=w416, y=w412) -> (x .or. y?=w413:bool)
        }
        n173 = call <vilib>:"Release Semaphore.vi"("error in (no error)"=w409, "semaphore"="Events Registered") -> ("error out"=w408:errorcluster)  [unwired: 4 in, 1 out]
        n174 = Bundle By Name(cluster=w411, "Panel Data.Hwnd"=w406) -> (w407:T6)
        n175 = Build Array (concatenate)(w404, "Update Global" ("String")) -> (w403:string[])
      }
      frame "-----Functions-----" {
      }
      frame "Update Global" {
        # "Take our data and write it to the global so the Parent has it."
        n176 = Unbundle By Name(w423) -> ("Panel Data.Panel VI Name"=w421:string, "Panel Data"=w420:T3)
        n177 = call "Panel Global Data.vi"("Method (Read All)"=Panel_Global_Methods."Write Panel Data", "error in (no error)"=w422, "Panel Data In"=w420, "Panel VI Name"=w421) -> ("error out"=w425:errorcluster)  [unwired: 4 in, 3 out]
      }
      frame "Hide VI" {
        w430 = TRUE ("Visible")
        # "Remove the Child from the subpanel, and replace it with a picture control the same size."
        n178 = Unbundle By Name(w446) -> ("Sub Panel"=w437:refnum<vi>, "VI Data.VI Ref"=w440:refnum<vi>)
        n179 = invoke on="Invoke Node" class="VI" method="FP.Get Image"(reference=w440, error in=w435, "image depth"=24 ("Image Depth")) -> (error out=w434:errorcluster, "image data"=w438:T14)  [unwired: 3 in, 4 out]
        n180 = invoke on="Invoke Node" class="SubPnl" method="Remove VI"(reference=w437, error in=w434) -> (reference out=w436:refnum<vi>, error out=w433:errorcluster)  [unwired: 1 in, 1 out]
        n181 = Unbundle By Name(w438) -> ("Rectangle.right"=w445:i16, "Rectangle.bottom"=w444:i16)
        n182 = property class="SubPnl"(reference=w436, error in=w433) -> (error out=w427:errorcluster, "Position"=w428:T2)  [unwired: 1 out]
        n183 = call <vilib>:"Draw Flattened Pixmap.vi"("image data"=w438) -> ("new picture"=→"2D Picture":picture)  [unwired: 8 in]
        n184 = property on="2D Picture" class="Pict"(error in=w427, "Position"=w428) -> (error out=w442:errorcluster)  [unwired: 1 in, 1 out]
        n185 = Bundle("right"=w445, "bottom"=w444) -> (w443:cluster{"right":i16, "bottom":i16})  [unwired: 1 in]
        n186 = property on="2D Picture" class="Pict"(error in=w442, "Draw Area Size"=w443) -> (error out=w441:errorcluster)  [unwired: 1 in, 1 out]
        n187 = Not(x=w430) -> (.not. x?=w429:bool)
        n188 = property on="Sub Panel" class="SubPnl"("Visible"=w429) -> ()  [unwired: 2 in, 2 out]
        n189 = property on="2D Picture" class="Pict"(error in=w441, "Visible"=w430) -> (error out=w431:errorcluster)  [unwired: 1 in, 1 out]
      }
      frame "Show VI" {
        # "Hide the picture control and insert the Child VI back into the subpanel."
        n190 = Unbundle By Name(w454) -> ("Sub Panel"=w455:refnum<vi>, "VI Data.VI Ref"=w453:refnum<vi>)
        n191 = property on="2D Picture" class="Pict"(error in=w450, "Visible"=FALSE) -> (error out=w449:errorcluster)  [unwired: 1 in, 1 out]
        n192 = invoke on="Invoke Node" class="SubPnl" method="Insert VI"(reference=w455, error in=w449, "VI Ref"=w453) -> (error out=w448:errorcluster)  [unwired: 1 in, 3 out]
        n193 = Bundle By Name(cluster=w454, "Saved Panel Size"=T5 {"Width"=0, "Height"=0}) -> (w452:T6)
      }
      frame "Allow Resize", "Disallow Resize" {
        # "Set the VI Properties to allow resize (or not) and modify the resize function within Windows, then redraw it.  \n\nWe do it this way because when a Panel VI is docked in the Parent, the resize only works if Windows draws thick boarders around it so we can drag it.  But if the Panel VI is undocked then changing the VI properties is all that is needed.  This will handle both cases by changing them both when needed."
        n194 = Unbundle By Name(w468) -> ("Panel Data.Hwnd"=w467:u32, "Panel Data.Docked?"=w458:bool, "Currently Resizeable?"=w463:bool)
        n195 = Equal?(x="Allow Resize", y=w466) -> (x = y?=w464:bool)
        n196 = And(x=w463, y=w464) -> (x .and. y?=w461:bool)
        n197 = case shown="False" w458 {
          tunnel: w461 -> [w473 _]
          tunnel: w460 -> [w472 w474]
          tunnel: [w471 w474] -> w459
          frame False {
            n198 = property class="VI"(error in=w472, "Front Panel.Resizeable"=w473) -> (error out=w471:errorcluster)  [unwired: 1 in, 1 out]
          }
          frame True {
          }
        }
        n199 = call "Allow Window Resize.vi"("error in (no error)"=w459, "Allow Resize?"=w461, "Hwnd"=w467) -> ("error out"=w469:errorcluster)  [unwired: 8 in]
        n200 = call "Redraw Window.vi"("error in (no error)"=w469, "Hwnd"=w467) -> ("error out"=w462:errorcluster)  [unwired: 9 in]
      }
      frame "Maximize Panel", "Minimize Panel" {
        # "WARNING this code is ugly....sorry."
        # "Hide the picture after the move."
        # "Set the pane color to match the top pane."
        # "Stop if error, movement complete, or movement is 0 pixels."
        # "Slide the window up or down logrithmicly so motion slows down approaching the move."
        n201 = Unbundle By Name(w476) -> ("Parent Hwnd"=w492:u32, "Panel Data.Hwnd"=w491:u32, "Panel Data.Docked?"=w480:bool)
        n202 = property class="VI"() -> ("Front Panel.PanelBounds"=w479:T12)  [unwired: 2 in, 2 out]
        n203 = case shown="\"Maximize Panel\", Default" w477 {
          tunnel: w476 -> [w521 w523]
          tunnel: [w520 w522] -> w502
          frame "Minimize Panel" {
            n204 = Unbundle By Name(w521) -> ("Reposition Offset.Top"=w520:i32)
          }
          frame "Maximize Panel", Default {
            n205 = Unbundle By Name(w523) -> ("Saved Panel Size.Height"=w522:u32)
            n206 = property on="Pane 2" class="Pane"("PaneColor"=u32 11776947) -> ()  [unwired: 2 in, 2 out]
            n207 = property on="2D Picture" class="Pict"("Visible"=TRUE) -> ()  [unwired: 2 in, 2 out]
          }
        }
        n208 = case shown="True" w480 {
          tunnel: w492 -> [_ w515]
          tunnel: w491 -> [_ w514]
          tunnel: [w512 w513] -> w484
          frame False {
            n209 = property class="VI"() -> ("Front Panel.PanelBounds"=w512:T12)  [unwired: 2 in, 2 out]
          }
          frame True {
            n210 = call "Get Child Coordinates.vi"("Child hWnd"=w514, "Parent hWnd"=w515) -> ("Relative"=w513:T13)  [unwired: 7 in, 2 out]
          }
        }
        n211 = call "Extract Window Origin and Size.vi"("window rect"=w479) -> ("window size"=w478:cluster{"width":i16, "height":i16})  [unwired: 1 out]
        n212 = Unbundle By Name(w484) -> ("left"=w483:i16, "top"=w482:i16)
        n213 = To Word Integer(number=w502) -> (16bit integer=w500:i16)
        n214 = Unbundle By Name(w478) -> ("width"=w489:i16, "height"=w490:i16)
        n215 = Add(x=w490, y=w482) -> (x+y=w486:i16)
        n216 = Add(x=w489, y=w483) -> (x+y=w487:i16)
        n217 = Bundle By Name(cluster=T10 {"left"=0, "top"=0, "right"=0, "bottom"=0} ("window rect"), "left"=w483, "top"=w482, "right"=w487, "bottom"=w486) -> (w485:T10)
        n218 = Unbundle By Name(w485) -> ("top"=w501:i16, "bottom"=w503:i16)
        n219 = Add(x=w500, y=w501) -> (x+y=w497:i16)
        n220 = for {
          N: 16 -> [_]
          tunnel: w497 -> [w537]
          tunnel: u32 40 ("Slide Delay (40)") -> [w536]
          shift-right: [w535] -> w494
          shift-left: w506 -> [w526]
          shift-right: [w529] -> _
          shift-left: w503 -> [w533]
          tunnel: w485 -> [w531]
          tunnel: [w527] -> w499
          tunnel: [w526] -> w498
          stop <- w534 stop-if-true
          n221 = Subtract(x=w533, y=w537) -> (x-y=w542:i16)
          n222 = Divide(x=w542, y=2) -> (x/y=w538:dbl)
          n223 = Negate(x=w538) -> (-x=w528:dbl)
          n224 = Add(x=w533, y=w528) -> (x+y=w530:dbl)
          n225 = Absolute Value(x=w528) -> (abs(x)=w540:dbl)
          n226 = To Word Integer(number=w530) -> (16bit integer=w529:i16)
          n227 = Round Toward -Infinity(1:w540) -> (0:w539:dbl)
          n228 = Equal To 0?(x=w539) -> (x = 0?=w527:bool)
          n229 = Bundle By Name(cluster=w531, "bottom"=w529) -> (w532:T10)
          n230 = property class="VI"(error in=w526, "Front Panel.PanelBounds"=w532) -> (error out=w535:errorcluster)  [unwired: 1 in, 1 out]
          n231 = case shown="No Error" w535 {
            tunnel: w536 -> [w543 _]
            frame No Error {
              n232 = Wait (ms)(milliseconds to wait=w543) -> ()  [unwired: 1 out]
            }
            frame Error {
            }
          }
          n233 = Compound Arithmetic op=OR(w535, w527) -> (w534:bool)
        }
        n234 = Bundle By Name(cluster=w485, "bottom"=w497) -> (w496:T10)
        n235 = case shown="\"Maximize Panel\", Default" w477 {
          tunnel: w499 -> [_ _]
          tunnel: [FALSE ("Visible") FALSE ("Visible")] -> w493
          frame "Maximize Panel", Default {
            n236 = property on="Sub Panel" class="SubPnl"("Visible"=TRUE) -> ()  [unwired: 2 in, 2 out]
            n237 = invoke on="Sub Panel" class="SubPnl" method="FitControlToPane"() -> ()  [unwired: 3 in, 3 out]
          }
          frame "Minimize Panel" {
            n238 = property on="Pane 2" class="Pane"("PaneColor"=u32 6845859) -> ()  [unwired: 2 in, 2 out]
          }
        }
        n239 = case shown="\"Minimize Panel\"" w477 {
          tunnel: w476 -> [w509 w511]
          tunnel: [w507 w511] -> w475
          frame "Minimize Panel" {
            n240 = property class="VI"() -> ("Front Panel.PanelBounds"=w510:T12)  [unwired: 2 in, 2 out]
            n241 = call "Extract Window Origin and Size.vi"("window rect"=w510) -> ("window size"=w508:cluster{"width":i16, "height":i16})  [unwired: 1 out]
            n242 = Bundle By Name(cluster=w509, "Saved Panel Size"=w508) -> (w507:T6)
          }
          frame "Maximize Panel", Default {
          }
        }
        n243 = call <vilib>:"Clear Errors.vi"("error in (no error)"=w494) -> ()  [unwired: 5 in, 2 out]
        n244 = property class="VI"(error in=w498, "Front Panel.PanelBounds"=w496) -> (error out=w495:errorcluster)  [unwired: 1 in, 1 out]
        n245 = property on="2D Picture" class="Pict"("Visible"=w493) -> ()  [unwired: 2 in, 2 out]
        n246 = call <vilib>:"Clear Errors.vi"("error in (no error)"=w495) -> ()  [unwired: 5 in, 2 out]
      }
      frame "Set Minimum Size" {
        n247 = property on="Pane 2" class="Pane"(error in=w545, "Minimum Pane Size"=T7 {"Horizontal"=200, "Vertical"=100}) -> (error out=w544:errorcluster)  [unwired: 1 in, 1 out]
      }
      frame "Notify Parent Dock" {
        # "Notify the parent that we docked.  This is needed because we may have docked it into a new tab."
        n248 = Unbundle By Name(w552) -> ("Panel Data.Docked?"=w549:bool, "Panel Data.Panel VI Name"=w554:string, "Dock Event"=w553:refnum<user-event>)
        n249 = case shown="True" w549 {
          tunnel: w554 -> [_ w560]
          tunnel: w553 -> [_ w561]
          tunnel: w551 -> [w556 w557]
          tunnel: [w556 w562] -> w550
          frame False {
          }
          frame True {
            n250 = Set Variant Attribute(Variant=variant ("variant"), name="Event Name" ("Tag"), value=w560, error in=w557) -> (Variant out=w564:variant, error out=w563:errorcluster)  [unwired: 1 out]
            n251 = Generate User Event(user event=w561, event data cluster=w564, error in=w563) -> (error out=w562:errorcluster)  [unwired: 1 in, 1 out]
          }
        }
      }
      frame "-----Development Errors-----" {
      }
      frame "Error" {
        n252 = case shown="\"Clear Error Cleanup\"" T11."Notify User Clear Error" ("Enum") {
          tunnel: w572 -> [w576 w581 w584]
          tunnel: [w575 w580 w585] -> w571
          tunnel: w569 -> [w574 w578 w582]
          tunnel: [w574 w577 w582] -> w570
          frame "Clear Error And Continue", Default {
            # "Clear error and continue"
            n253 = call <vilib>:"Clear Errors.vi"("error in (no error)"=w576) -> ("error out"=w575:errorcluster)  [unwired: 5 in, 1 out]
          }
          frame "Clear Error Cleanup" {
            # "Clear the error then run Cleanup."
            n254 = call <vilib>:"Clear Errors.vi"("error in (no error)"=w581) -> ("error out"=w580:errorcluster)  [unwired: 5 in, 1 out]
            n255 = Build Array (concatenate)(w578, "Cleanup" ("Element to Add")) -> (w577:string[])
          }
          frame "Notify User Clear Error" {
            # "Notify the user of the error then continue."
            n256 = call <vilib>:"Simple Error Handler.vi"("error in (no error)"=w584) -> ("error out"=w583:errorcluster)  [unwired: 4 in, 4 out]
            n257 = call <vilib>:"Clear Errors.vi"("error in (no error)"=w583) -> ("error out"=w585:errorcluster)  [unwired: 5 in, 1 out]
          }
        }
      }
      frame "Unhandled Case", Default {
        # "Notify the user of the unhandled case then continue."
        n258 = property class="VI"(error in=w587) -> (error out=w586:errorcluster, "Name"=w588:string)  [unwired: 1 in, 1 out]
        n259 = Format Into String(format string="Error:  Unhandled case\n\n%s\n\nIn VI %s", w589, w588) -> (resulting string=w590:string)  [unwired: 2 in, 1 out]
        n260 = One Button Dialog(message=w590) -> ()  [unwired: 1 in, 1 out]
      }
      frame "-----Exit Operations-----" {
      }
      frame "Cleanup" {
        # "When a graceful close operation is called we want to unregister for the events, then exit."
        n261 = Build Array (concatenate)(w598, string[] ["Quit Child VI", "Unregister Events", "Exit"]) -> (w597:string[])
      }
      frame "Quit Child VI" {
        w609 = "Quit" ("Event Name")
        # "Generate the Quit Event telling the Child VI to stop."
        n262 = Unbundle By Name(w608) -> ("VI Data.VI Ref"=w602:refnum<vi>, "VI Data.Events Variant"=w607:variant)
        n263 = call "Get User Event from Event Name.vi"("error in (no error)"=w605, "Event Data"=w607, "Event Name (Quit)"=w609) -> ("error out"=w606:errorcluster, "User Event out"=w610:refnum<user-event>)  [unwired: 7 in]
        n264 = call "Fire Event.vi"("Event Name"=w609, "error in (no error)"=w606, "User Event In"=w610) -> ("error out"=w604:errorcluster)  [unwired: 7 in, 1 out]
        n265 = Close Reference(reference=w602, error in (no error)=w604) -> (error out=w603:errorcluster)
      }
      frame "Unregister Events" {
        n266 = Unbundle By Name(w615) -> ("Event Ref"=w614:refnum<event-registration>)
        n267 = Unregister For Events(event registration refnum=w614, error in=w613) -> (error out=w612:errorcluster)
      }
      frame "Exit" {
        # "Code in this case will execute once on exit."
      }
    }
  }
  "error out" <- w2
